vi "EbN0required.vi"(1 "Modulation":string(combo)) -> (0 "Eb/N0 (dB) required for BER=10-4":dbl)   [LabVIEW 2015]
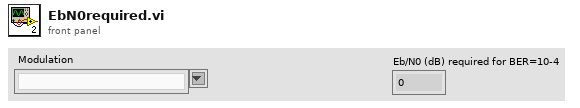
[diagram p1: front panel]
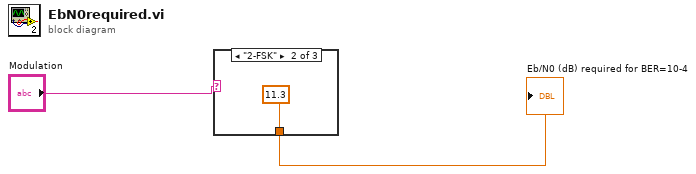
[diagram p0: block diagram]
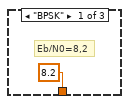
[diagram p2: hidden frame]
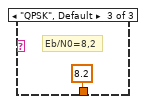
[diagram p3: hidden frame]
diagram:
  n1 = case shown="\"2-FSK\"" "Modulation" {
    tunnel: [8.2 11.3 8.2] -> w2
    frame "BPSK" {
      # "Eb/N0=8,2"
    }
    frame "2-FSK" {
    }
    frame "QPSK", Default {
      # "Eb/N0=8,2"
    }
  }
  "Eb/N0 (dB) required for BER=10-4" <- w2
